vi "Format Links Info for Table Display.vi"(10 "Remove module Name From First Column (F)":bool, 11 "Links Info":T1[](array[typedef])) -> (3 "Table Content":string[][](array[string]))   [LabVIEW 2021, in "TAF Proj Document Type.lvlib" / "Dqmh Module.lvclass"]
uses:
  <vilib>/Wovalab/AntiDoc/Document Type/Add-ons/LabVIEW TAF Project/Dqmh Module/Dqmh Module.lvclass
  <vilib>/Wovalab/AntiDoc/Document Type/Add-ons/LabVIEW TAF Project/Dqmh Module/Event Callers--cluster.ctl
  <vilib>/Wovalab/AntiDoc/Document Type/Add-ons/LabVIEW TAF Project/TAF Proj Document Type.lvlib
  <vilib>/Wovalab/AntiDoc/Utilities/Utilities.lvlib
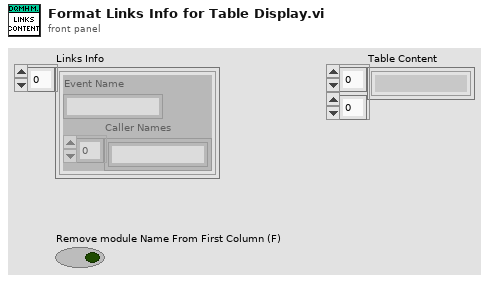
[diagram p1: front panel]
types:
  T1 = typedef "TAF Proj Document Type.lvlib/Dqmh Module.lvclass/Event Callers--cluster.ctl" = cluster{"Event Name":string, "Caller Names":string[]}
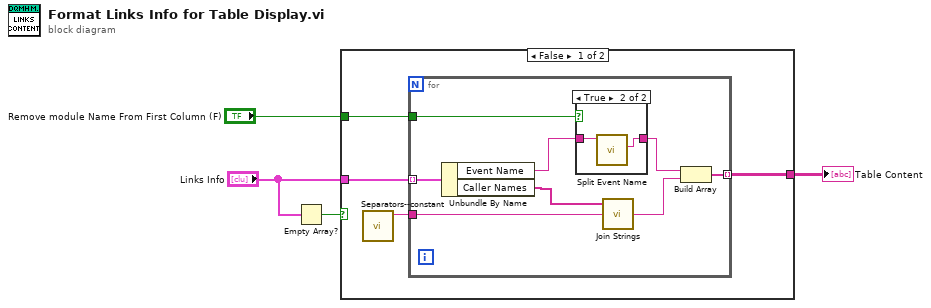
[diagram p0: block diagram]
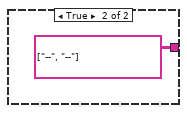
[diagram p3: hidden frame]
diagram:
  n1 = Empty Array?(array="Links Info") -> (empty?=w2:bool)
  n2 = case shown="False" w2 {
    tunnel: [w8 string[][] [["--", "--"]]] -> w4
    tunnel: "Links Info" -> [w7 _]
    tunnel: "Remove module Name From First Column (F)" -> [w6 _]
    frame False {
      n3 = call <vilib>:"Separators--constant.vi"() -> ("Caller Separator"=w5:string)  [unwired: 10 in, 1 out]
      n4 = for {
        tunnel: w7 -> [w16] mode=indexing
        tunnel: w5 -> [w14]
        tunnel: [w12] -> w8 mode=indexing
        tunnel: w6 -> [w9]
        n5 = Unbundle By Name(w16) -> ("Event Name"=w11:string, "Caller Names"=w15:string[])
        n6 = case shown="True" w9 {
          tunnel: w11 -> [w17 w19]
          tunnel: [w17 w18] -> w10
          frame False {
          }
          frame True {
            n7 = call <vilib>:"Split Event Name.vi"("Event Name"=w19) -> ("Vi Name"=w18:string)  [unwired: 8 in, 2 out]
          }
        }
        n8 = call <vilib>:"Join Strings.vi"("Separator (,)"=w14, "Strings In"=w15) -> ("String"=w13:string)  [unwired: 1 in]
        n9 = Build Array(w10, w13) -> (w12:string[])
      }
    }
    frame True {
    }
  }
  "Table Content" <- w4
